vi "Modra-StereoMadness.vi"(11 "NXT/EV3":T1) -> (3 "NXT/EV3 2":T1)   [LabVIEW 2016]
uses:
  <vilib>/NXT/Subs/LVHSConnector.ctl
  <vilib>/NXT/LegoClasses/BrickReference/BrickReference.lvclass
  <vilib>/NXT/Dual Mode Library/Display/drawText_Center.vi
  <vilib>/NXT/Dual Mode Library/Sound/PlayC.vi
  <vilib>/NXT/Dual Mode Library/Sound/PlayG.vi
  <vilib>/NXT/Dual Mode Library/Sound/PlayD.vi
  <vilib>/NXT/Dual Mode Library/Sound/PlayA.vi
  <vilib>/NXT/Dual Mode Library/Sound/PlayE.vi
  <vilib>/NXT/Dual Mode Library/Sound/PlayF.vi
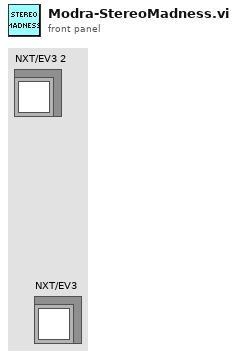
[diagram p1: front panel]
types:
  T1 = typedef "LVHSConnector.ctl" = refnum<class "BrickReference.lvclass">
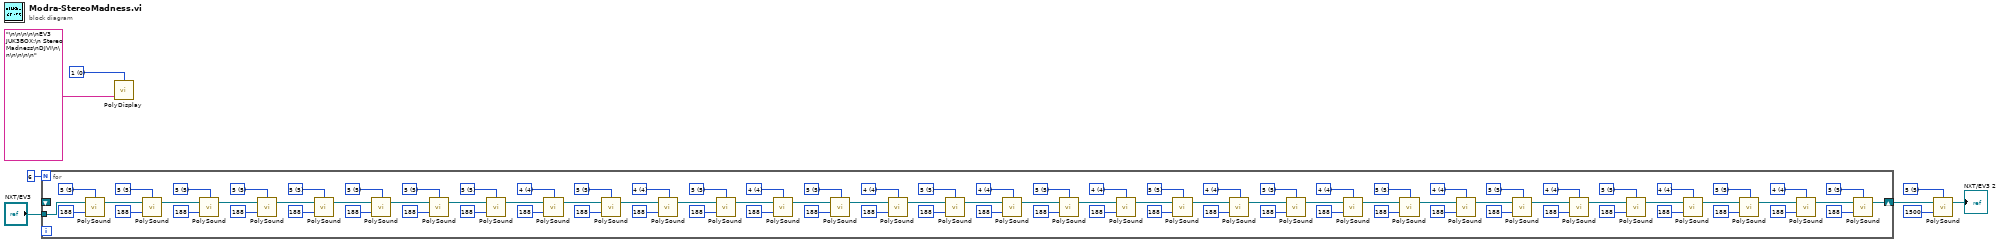
[diagram p0: block diagram]
diagram:
  w3 = u16 5 items=["3"=3, "4"=4, "5"=5, "6"=6, "7"=7] ("Octave")
  w7 = i16 0 items=["1", "2", "3", "4", "5", "6", "7", "8", "9", "10", "11", "12"] ("Line")
  n1 = for {
    N: 6 -> [_]
    shift-right: [w10] -> w2
    shift-left: _ -> [_]
    tunnel: "NXT/EV3" -> [w9]
    w27 = u16 4 items=["3"=3, "4"=4, "5"=5, "6"=6, "7"=7] ("Octave")
    w29 = u16 5 items=["3"=3, "4"=4, "5"=5, "6"=6, "7"=7] ("Octave")
    w26 = u16 4 items=["3"=3, "4"=4, "5"=5, "6"=6, "7"=7] ("Octave")
    w24 = u16 5 items=["3"=3, "4"=4, "5"=5, "6"=6, "7"=7] ("Octave")
    w17 = u16 4 items=["3"=3, "4"=4, "5"=5, "6"=6, "7"=7] ("Octave")
    w19 = u16 5 items=["3"=3, "4"=4, "5"=5, "6"=6, "7"=7] ("Octave")
    w16 = u16 4 items=["3"=3, "4"=4, "5"=5, "6"=6, "7"=7] ("Octave")
    w14 = u16 5 items=["3"=3, "4"=4, "5"=5, "6"=6, "7"=7] ("Octave")
    w43 = u16 4 items=["3"=3, "4"=4, "5"=5, "6"=6, "7"=7] ("Octave")
    w41 = u16 5 items=["3"=3, "4"=4, "5"=5, "6"=6, "7"=7] ("Octave")
    w44 = u16 4 items=["3"=3, "4"=4, "5"=5, "6"=6, "7"=7] ("Octave")
    w46 = u16 5 items=["3"=3, "4"=4, "5"=5, "6"=6, "7"=7] ("Octave")
    w53 = u16 4 items=["3"=3, "4"=4, "5"=5, "6"=6, "7"=7] ("Octave")
    w51 = u16 5 items=["3"=3, "4"=4, "5"=5, "6"=6, "7"=7] ("Octave")
    w54 = u16 4 items=["3"=3, "4"=4, "5"=5, "6"=6, "7"=7] ("Octave")
    w56 = u16 5 items=["3"=3, "4"=4, "5"=5, "6"=6, "7"=7] ("Octave")
    w75 = u16 4 items=["3"=3, "4"=4, "5"=5, "6"=6, "7"=7] ("Octave")
    w77 = u16 5 items=["3"=3, "4"=4, "5"=5, "6"=6, "7"=7] ("Octave")
    w74 = u16 4 items=["3"=3, "4"=4, "5"=5, "6"=6, "7"=7] ("Octave")
    w72 = u16 5 items=["3"=3, "4"=4, "5"=5, "6"=6, "7"=7] ("Octave")
    w65 = u16 4 items=["3"=3, "4"=4, "5"=5, "6"=6, "7"=7] ("Octave")
    w67 = u16 5 items=["3"=3, "4"=4, "5"=5, "6"=6, "7"=7] ("Octave")
    w64 = u16 4 items=["3"=3, "4"=4, "5"=5, "6"=6, "7"=7] ("Octave")
    w62 = u16 5 items=["3"=3, "4"=4, "5"=5, "6"=6, "7"=7] ("Octave")
    w90 = u16 5 items=["3"=3, "4"=4, "5"=5, "6"=6, "7"=7] ("Octave")
    w88 = u16 5 items=["3"=3, "4"=4, "5"=5, "6"=6, "7"=7] ("Octave")
    w91 = u16 5 items=["3"=3, "4"=4, "5"=5, "6"=6, "7"=7] ("Octave")
    w93 = u16 5 items=["3"=3, "4"=4, "5"=5, "6"=6, "7"=7] ("Octave")
    w100 = u16 5 items=["3"=3, "4"=4, "5"=5, "6"=6, "7"=7] ("Octave")
    w98 = u16 5 items=["3"=3, "4"=4, "5"=5, "6"=6, "7"=7] ("Octave")
    w101 = u16 5 items=["3"=3, "4"=4, "5"=5, "6"=6, "7"=7] ("Octave")
    w103 = u16 5 items=["3"=3, "4"=4, "5"=5, "6"=6, "7"=7] ("Octave")
    n2 = call-poly <vilib>:"PolySound.vi"("Duration (500 ms)"=u16 188, "NXT/EV3"=w9, "Octave"=w101) -> ("NXT/EV3"=w102:T1)  [unwired: 1 in]
    n3 = call-poly <vilib>:"PolySound.vi"("Duration (500 ms)"=u16 188, "NXT/EV3"=w102, "Octave"=w103) -> ("NXT/EV3"=w85:T1)  [unwired: 1 in]
    n4 = call-poly <vilib>:"PolySound.vi"("Duration (500 ms)"=u16 188, "NXT/EV3"=w85, "Octave"=w100) -> ("NXT/EV3"=w99:T1)  [unwired: 1 in]
    n5 = call-poly <vilib>:"PolySound.vi"("Duration (500 ms)"=u16 188, "NXT/EV3"=w99, "Octave"=w98) -> ("NXT/EV3"=w84:T1)  [unwired: 1 in]
    n6 = call-poly <vilib>:"PolySound.vi"("Duration (500 ms)"=u16 188, "NXT/EV3"=w84, "Octave"=w91) -> ("NXT/EV3"=w92:T1)  [unwired: 1 in]
    n7 = call-poly <vilib>:"PolySound.vi"("Duration (500 ms)"=u16 188, "NXT/EV3"=w92, "Octave"=w93) -> ("NXT/EV3"=w83:T1)  [unwired: 1 in]
    n8 = call-poly <vilib>:"PolySound.vi"("Duration (500 ms)"=u16 188, "NXT/EV3"=w83, "Octave"=w90) -> ("NXT/EV3"=w89:T1)  [unwired: 1 in]
    n9 = call-poly <vilib>:"PolySound.vi"("Duration (500 ms)"=u16 188, "NXT/EV3"=w89, "Octave"=w88) -> ("NXT/EV3"=w59:T1)  [unwired: 1 in]
    n10 = call-poly <vilib>:"PolySound.vi"("Duration (500 ms)"=u16 188, "NXT/EV3"=w59, "Octave"=w64) -> ("NXT/EV3"=w63:T1)  [unwired: 1 in]
    n11 = call-poly <vilib>:"PolySound.vi"("Duration (500 ms)"=u16 188, "NXT/EV3"=w63, "Octave"=w62) -> ("NXT/EV3"=w80:T1)  [unwired: 1 in]
    n12 = call-poly <vilib>:"PolySound.vi"("Duration (500 ms)"=u16 188, "NXT/EV3"=w80, "Octave"=w65) -> ("NXT/EV3"=w66:T1)  [unwired: 1 in]
    n13 = call-poly <vilib>:"PolySound.vi"("Duration (500 ms)"=u16 188, "NXT/EV3"=w66, "Octave"=w67) -> ("NXT/EV3"=w81:T1)  [unwired: 1 in]
    n14 = call-poly <vilib>:"PolySound.vi"("Duration (500 ms)"=u16 188, "NXT/EV3"=w81, "Octave"=w74) -> ("NXT/EV3"=w73:T1)  [unwired: 1 in]
    n15 = call-poly <vilib>:"PolySound.vi"("Duration (500 ms)"=u16 188, "NXT/EV3"=w73, "Octave"=w72) -> ("NXT/EV3"=w82:T1)  [unwired: 1 in]
    n16 = call-poly <vilib>:"PolySound.vi"("Duration (500 ms)"=u16 188, "NXT/EV3"=w82, "Octave"=w75) -> ("NXT/EV3"=w76:T1)  [unwired: 1 in]
    n17 = call-poly <vilib>:"PolySound.vi"("Duration (500 ms)"=u16 188, "NXT/EV3"=w76, "Octave"=w77) -> ("NXT/EV3"=w35:T1)  [unwired: 1 in]
    n18 = call-poly <vilib>:"PolySound.vi"("Duration (500 ms)"=u16 188, "NXT/EV3"=w35, "Octave"=w54) -> ("NXT/EV3"=w55:T1)  [unwired: 1 in]
    n19 = call-poly <vilib>:"PolySound.vi"("Duration (500 ms)"=u16 188, "NXT/EV3"=w55, "Octave"=w56) -> ("NXT/EV3"=w38:T1)  [unwired: 1 in]
    n20 = call-poly <vilib>:"PolySound.vi"("Duration (500 ms)"=u16 188, "NXT/EV3"=w38, "Octave"=w53) -> ("NXT/EV3"=w52:T1)  [unwired: 1 in]
    n21 = call-poly <vilib>:"PolySound.vi"("Duration (500 ms)"=u16 188, "NXT/EV3"=w52, "Octave"=w51) -> ("NXT/EV3"=w37:T1)  [unwired: 1 in]
    n22 = call-poly <vilib>:"PolySound.vi"("Duration (500 ms)"=u16 188, "NXT/EV3"=w37, "Octave"=w44) -> ("NXT/EV3"=w45:T1)  [unwired: 1 in]
    n23 = call-poly <vilib>:"PolySound.vi"("Duration (500 ms)"=u16 188, "NXT/EV3"=w45, "Octave"=w46) -> ("NXT/EV3"=w36:T1)  [unwired: 1 in]
    n24 = call-poly <vilib>:"PolySound.vi"("Duration (500 ms)"=u16 188, "NXT/EV3"=w36, "Octave"=w43) -> ("NXT/EV3"=w42:T1)  [unwired: 1 in]
    n25 = call-poly <vilib>:"PolySound.vi"("Duration (500 ms)"=u16 188, "NXT/EV3"=w42, "Octave"=w41) -> ("NXT/EV3"=w11:T1)  [unwired: 1 in]
    n26 = call-poly <vilib>:"PolySound.vi"("Duration (500 ms)"=u16 188, "NXT/EV3"=w11, "Octave"=w16) -> ("NXT/EV3"=w15:T1)  [unwired: 1 in]
    n27 = call-poly <vilib>:"PolySound.vi"("Duration (500 ms)"=u16 188, "NXT/EV3"=w15, "Octave"=w14) -> ("NXT/EV3"=w32:T1)  [unwired: 1 in]
    n28 = call-poly <vilib>:"PolySound.vi"("Duration (500 ms)"=u16 188, "NXT/EV3"=w32, "Octave"=w17) -> ("NXT/EV3"=w18:T1)  [unwired: 1 in]
    n29 = call-poly <vilib>:"PolySound.vi"("Duration (500 ms)"=u16 188, "NXT/EV3"=w18, "Octave"=w19) -> ("NXT/EV3"=w33:T1)  [unwired: 1 in]
    n30 = call-poly <vilib>:"PolySound.vi"("Duration (500 ms)"=u16 188, "NXT/EV3"=w33, "Octave"=w26) -> ("NXT/EV3"=w25:T1)  [unwired: 1 in]
    n31 = call-poly <vilib>:"PolySound.vi"("Duration (500 ms)"=u16 188, "NXT/EV3"=w25, "Octave"=w24) -> ("NXT/EV3"=w34:T1)  [unwired: 1 in]
    n32 = call-poly <vilib>:"PolySound.vi"("Duration (500 ms)"=u16 188, "NXT/EV3"=w34, "Octave"=w27) -> ("NXT/EV3"=w28:T1)  [unwired: 1 in]
    n33 = call-poly <vilib>:"PolySound.vi"("Duration (500 ms)"=u16 188, "NXT/EV3"=w28, "Octave"=w29) -> ("NXT/EV3"=w10:T1)  [unwired: 1 in]
  }
  n34 = call-poly <vilib>:"PolyDisplay.vi"("Text"="\n\n\n\n\nEV3 JUK3BOX:\n Stereo Madness\nDJVI\n\n\n\n\n\n", "Line"=w7) -> ()  [unwired: 2 in, 1 out]
  n35 = call-poly <vilib>:"PolySound.vi"("Duration (500 ms)"=u16 1500, "NXT/EV3"=w2, "Octave"=w3) -> ("NXT/EV3"=→"NXT/EV3 2":T1)  [unwired: 1 in]
